vi "High G csv string constants.vi"(11 "error in (no error)":errorcluster) -> (6 "Header":string, 8 "Delimiter":string, 10 "Format string":string, 15 "error out":errorcluster)   [LabVIEW 2011]
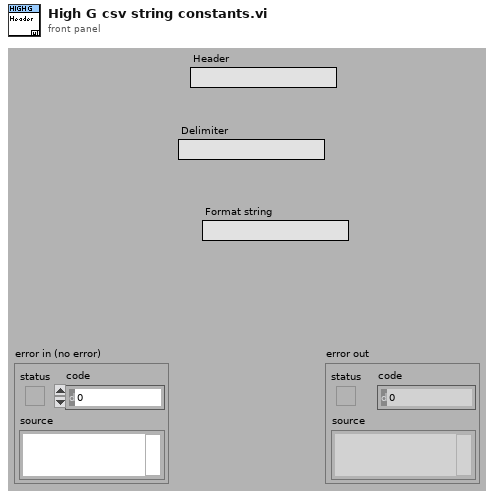
[diagram p1: front panel]
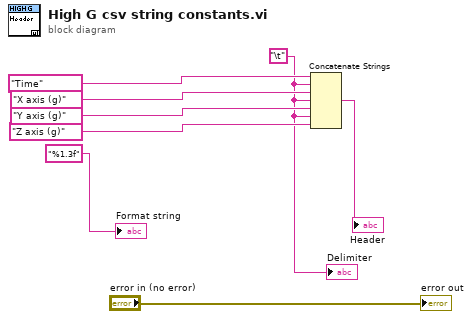
[diagram p0: block diagram]
diagram:
  w2 = "\t"
  n1 = Concatenate Strings("Time" ("string"), w2, "X axis (g)" ("string"), w2, "Y axis (g)" ("string"), w2, "Z axis (g)" ("string")) -> (→"Header":string)
  "Format string" <- "%1.3f" ("format string")
  "Delimiter" <- w2
  "error out" <- "error in (no error)"
